vi "Unit definition.vi"() -> (3 "Array":T1(array[cluster]))   [LabVIEW 2011]
uses:
  Quantity enum.ctl
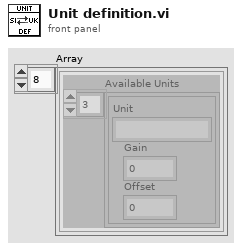
[diagram p1: front panel]
types:
  T1 = cluster{"Available Units":cluster{"Unit":string, "Gain":dbl, "Offset":dbl}[]}[]
  T2 = typedef "Quantity enum.ctl" = enum16{"NA", "Acceleration", "Angle", "Current", "Force", "Distance", "Pressure", "Resistance", "Rotational Speed", "Speed", "Temperature", "Tension", "Torque", "Voltage", "Weight"}
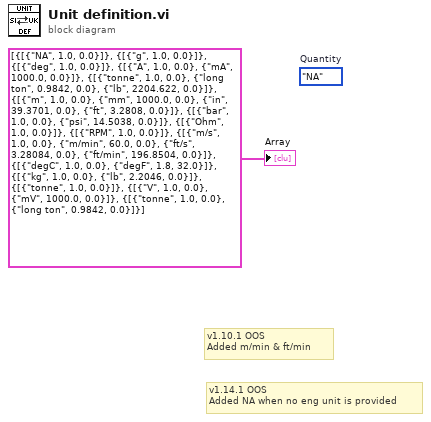
[diagram p0: block diagram]
diagram:
  (unwired) Quantity_enum."NA"  # Quantity
  # "v1.14.1 OOS\nAdded NA when no eng unit is provided"
  # "v1.10.1 OOS\nAdded m/min & ft/min"
  "Array" <- T1 [{"Available Units"=[{"Unit"="NA", "Gain"=1.0, "Offset"=0.0}]}, {"Available Units"=[{"Unit"="g", "Gain"=1.0, "Offset"=0.0}]}, {"Available Units"=[{"Unit"="deg", "Gain"=1.0, "Offset"=0.0}]}, {"Available Units"=[{"Unit"="A", "Gain"=1.0, "Offset"=0.0}, {"Unit"="mA", "Gain"=1000.0, "Offset"=0.0}]}, {"Available Units"=[{"Unit"="tonne", "Gain"=1.0, "Offset"=0.0}, {"Unit"="long ton", "Gain"=0.9842, "Offset"=0.0}, {"Unit"="lb", "Gain"=2204.622, "Offset"=0.0}]}, {"Available Units"=[{"Unit"="m", "Gain"=1.0, "Offset"=0.0}, {"Unit"="mm", "Gain"=1000.0, "Offset"=0.0}, {"Unit"="in", "Gain"=39.3701, "Offset"=0.0}, {"Unit"="ft", "Gain"=3.2808, "Offset"=0.0}]}, {"Available Units"=[{"Unit"="bar", "Gain"=1.0, "Offset"=0.0}, {"Unit"="psi", "Gain"=14.5038, "Offset"=0.0}]}, {"Available Units"=[{"Unit"="Ohm", "Gain"=1.0, "Offset"=0.0}]}, {"Available Units"=[{"Unit"="RPM", "Gain"=1.0, "Offset"=0.0}]}, {"Available Units"=[{"Unit"="m/s", "Gain"=1.0, "Offset"=0.0}, {"Unit"="m/min", "Gain"=60.0, "Offset"=0.0}, {"Unit"="ft/s", "Gain"=3.28084, "Offset"=0.0}, {"Unit"="ft/min", "Gain"=196.8504, "Offset"=0.0}]}, {"Available Units"=[{"Unit"="degC", "Gain"=1.0, "Offset"=0.0}, {"Unit"="degF", "Gain"=1.8, "Offset"=32.0}]}, {"Available Units"=[{"Unit"="kg", "Gain"=1.0, "Offset"=0.0}, {"Unit"="lb", "Gain"=2.2046, "Offset"=0.0}]}, {"Available Units"=[{"Unit"="tonne", "Gain"=1.0, "Offset"=0.0}]}, {"Available Units"=[{"Unit"="V", "Gain"=1.0, "Offset"=0.0}, {"Unit"="mV", "Gain"=1000.0, "Offset"=0.0}]}, {"Available Units"=[{"Unit"="tonne", "Gain"=1.0, "Offset"=0.0}, {"Unit"="long ton", "Gain"=0.9842, "Offset"=0.0}]}]
